vi "FlattenTOAPsetup.vi"() -> ()   [LabVIEW 2022 SP3]
uses:
  TOAPspecs.ctl
panel:
  out "xml string":string
  in  "outerClusterName":T1={"textOrigin"={"x"=0, "y"=0}, "textAlignment"={"horizontal"=enum."left", "vertical"=enum."top"}, "fontColour"={"text color"=12632256, "BG color"=0, "orientation "=enum."None"}, "fontChoice"=enum."User-specified Font", "userFont"={"Font Name:"="Helvetica", "Size"=18, "Strikeout?"=FALSE, "Italic?"=FALSE, "Underline?"=FALSE, "Outline?"=FALSE, "Shadow?"=FALSE, "Bold?"=FALSE}}
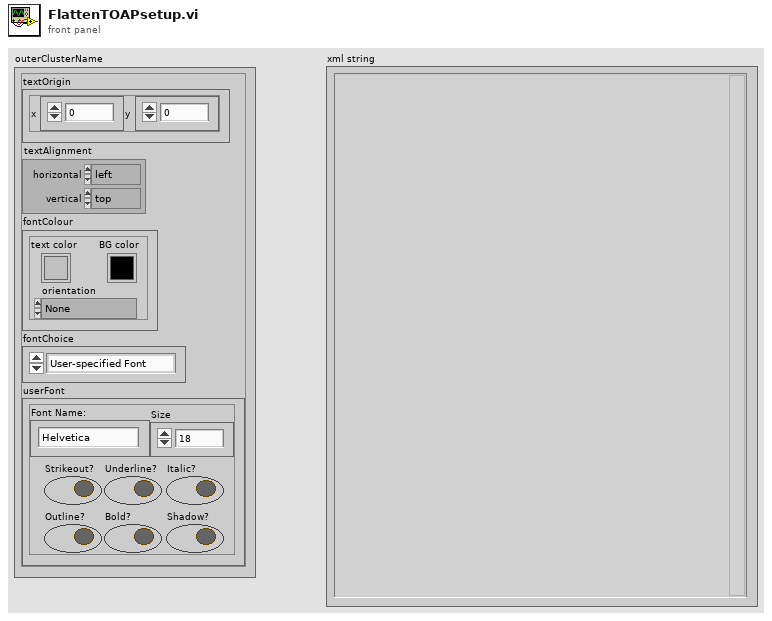
[diagram p1: front panel]
types:
  T1 = typedef "TOAPspecs.ctl" = cluster{"textOrigin":cluster{"x":i16, "y":i16}, "textAlignment":cluster{"horizontal":enum16{"left", "center", "right"}, "vertical":enum16{"top", "center", "bottom"}}, "fontColour":cluster{"text color":u32, "BG color":u32, "orientation ":enum16{"None", "Stacked", "Clockwise", "Counterclockwise"}}, "fontChoice":enum16{"User-specified Font", "Application Font", "System Font", "Dialog Font"}, "userFont":cluster{"Font Name:":string, "Size":i16, "Strikeout?":bool, "Italic?":bool, "Underline?":bool, "Outline?":bool, "Shadow?":bool, "Bold?":bool}}
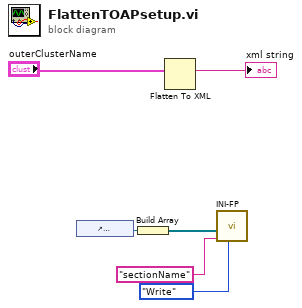
[diagram p0: block diagram]
diagram:
  n1 = control-ref of="outerClusterName"() -> (w4:refnum<vi>)
  n2 = Build Array(w4) -> (w3:refnum<vi>[])
  n3 = Flatten To XML(6:"outerClusterName") -> (2:→"xml string":string)
  n4 = call "INI-FP.vi"("Mode"=enum16{"Read", "Write"}."Write", "section"="sectionName", "Controls[]"=w3) -> ()  [unwired: 7 in, 2 out]
